vi "Get Dichotomie.vi"(11 "Ball-Ball in":refnum<class "Ball-Ball.lvclass">) -> (2 "Dichotomie out":i32)   [LabVIEW 2024, in "Ball-Ball.lvclass"]
doc: "MIT Licence\nCopyright (c) 2024 David Grollier"
uses:
  Ball-Ball.lvclass
  Collision.lvclass
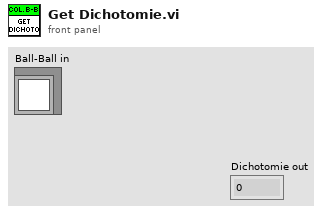
[diagram p1: front panel]
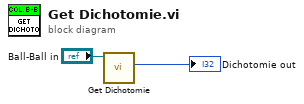
[diagram p0: block diagram]
diagram:
  n1 = call-parent "Get Dichotomie.vi"("Collision in"="Ball-Ball in") -> ("Dichotomie out"=→"Dichotomie out":i32)  [unwired: 10 in]
